vi "WPI_JoystickSetOutputs.vi"(6 "Outputs":bool[](array[boolean]), 8 "error in (no error)":errorcluster, 9 "Right Rumble":sgl, 10 "Left Rumble":sgl, 11 "JoystickDevRef":T1) -> (0 "error out":errorcluster, 3 "JoystickDevRef":T1)   [LabVIEW 2017]
doc: "Updates rumble and driven outputs for a USB joystick device that you specify.\n\nThis software is licensed. Open the labview\\readme\\WPI Robotics Library Open Source License.txt file for more information."
uses:
  <vilib>/Rock Robotics/WPI/Joystick/WPI_JoystickDevRef.ctl
  <vilib>/Rock Robotics/WPI/Joystick/WPI_JoystickDeviceEnum.ctl
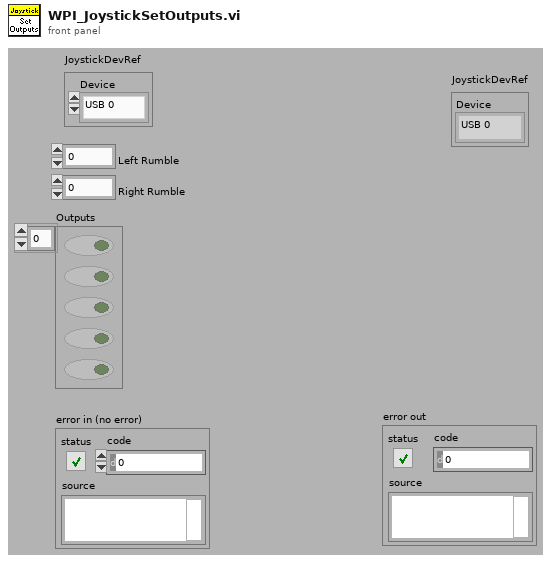
[diagram p1: front panel]
types:
  T1 = typedef "WPI_JoystickDevRef.ctl" = cluster{"Device":T2}
  T2 = typedef "WPI_JoystickDeviceEnum.ctl" = enum16{"USB 0", "USB 1", "USB 2", "USB 3", "USB 4", "USB 5"}
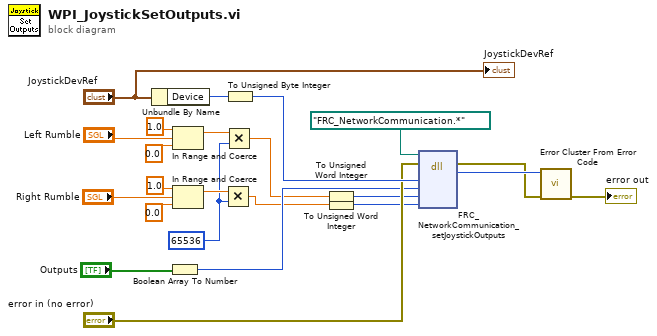
[diagram p0: block diagram]
diagram:
  w5 = 65536
  n1 = Unbundle By Name("JoystickDevRef") -> ("Device"=w14:T2)
  n2 = Boolean Array To Number(Boolean array="Outputs") -> (number=w8:u32)
  n3 = In Range and Coerce(upper limit=1.0, x="Left Rumble", lower limit=0.0) -> (coerced(x)=w6:dbl)  [unwired: 1 out]
  n4 = In Range and Coerce(upper limit=1.0, x="Right Rumble", lower limit=0.0) -> (coerced(x)=w7:dbl)  [unwired: 1 out]
  n5 = Multiply(x=w7, y=w5) -> (x*y=w3:dbl)
  n6 = Multiply(x=w6, y=w5) -> (x*y=w4:dbl)
  n7 = To Unsigned Byte Integer(number=w14) -> (unsigned 8bit integer=w16:u8)
  n8 = To Unsigned Word Integer(number=w4) -> (unsigned 16bit integer=w2:u16)
  n9 = To Unsigned Word Integer(number=w3) -> (unsigned 16bit integer=w1:u16)
  n10 = dll-call lib="?" fn="FRC_NetworkCommunication_setJoystickOutputs"(path in=path "FRC_NetworkCommunication.*", error in="error in (no error)", "joystickNum"=w16, "hidOutputs"=w8, "leftRumble"=w2, "rightRumble"=w1) -> (error out=w11:errorcluster, "return type"=w12:i32)  [unwired: 5 in, 1 out]
  n11 = call <vilib>:"Error Cluster From Error Code.vi"("error in (no error)"=w11, "error code (0)"=w12) -> ("error out"=→"error out":errorcluster)  [unwired: 7 in]
  "JoystickDevRef" <- "JoystickDevRef"
